vi "SendQuery.vi"(8 "error in (no error)":errorcluster, 11 "TCPComm in":refnum<class "TCPCommClass.lvclass">) -> (0 "error out":errorcluster, 3 "TCPComm out":refnum<class "TCPCommClass.lvclass">)   [LabVIEW 2013, in "TCPCommClass.lvclass"]
uses:
  TCPCommClass.lvclass
  TCPCommClass.lvclass/TCPCommClass.ctl
panel:
  in  "Initial byte timeout ms (1000)":i32=1000
  in  "old tcp":bool
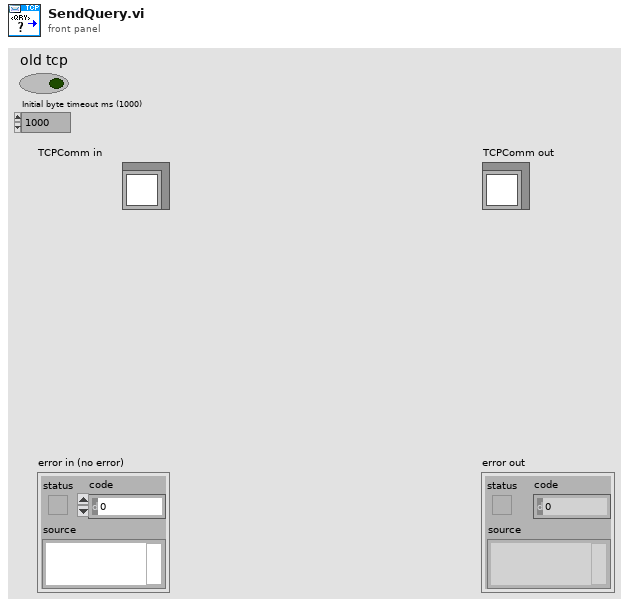
[diagram p1: front panel]
types:
  T1 = enum16{"Standard", "Buffered", "CRLF", "Immediate"}
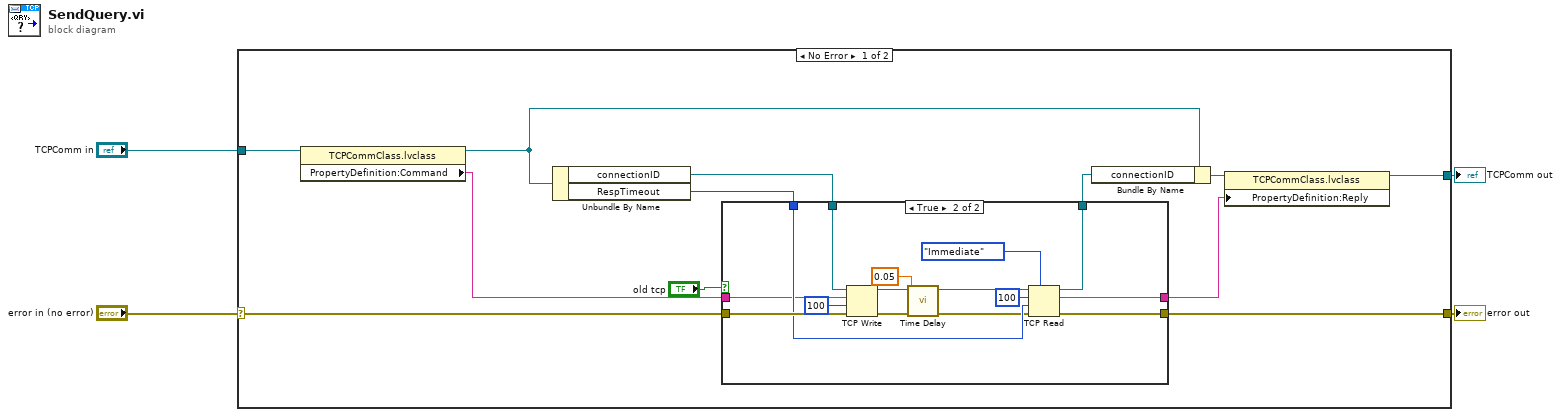
[diagram p0: block diagram]
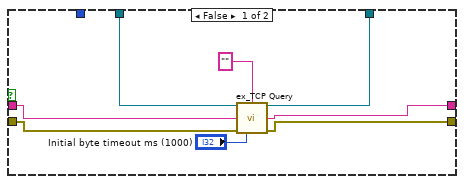
[diagram p2: hidden frame]
diagram:
  n1 = case shown="No Error" "error in (no error)" {
    selector: "error in (no error)" -> [w16 w40]
    tunnel: [w15 w40] -> w3
    tunnel: [w8 w39] -> w1
    tunnel: "TCPComm in" -> [w11 w39]
    frame No Error {
      n2 = property class="TCPCommClass.lvclass"(reference=w11) -> (reference out=w10:refnum<class "TCPCommClass.lvclass">, "PropertyDefinition:Command"=w6:string)  [unwired: 1 in, 1 out]
      n3 = Unbundle By Name(w10) -> ("connectionID"=w13:refnum<k5>, "RespTimeout"=w12:i32)
      n4 = case shown="True" "old tcp" {
        tunnel: w16 -> [w20 w34]
        tunnel: [w19 w33] -> w15
        tunnel: [w22 w32] -> w14
        tunnel: w13 -> [w23 w31]
        tunnel: w12 -> [_ w30]
        tunnel: [w18 w29] -> w7
        tunnel: w6 -> [w21 w28]
        frame False {
          n5 = call "ex_TCP Query.vi"("TCP Network Connection in"=w23, "Termination character"="", "Query string"=w21, "error in (no error)"=w20, "Initial byte timeout ms (1000)"="Initial byte timeout ms (1000)") -> ("TCP Network Connection out"=w22:refnum<k5>, "Message data out"=w18:string, "error out"=w19:errorcluster)  [unwired: 7 in, 1 out]
        }
        frame True {
          n6 = TCP Write(connection ID=w31, data in=w28, error in (no error)=w34, 9:100 ("bytes to read")) -> (connection ID out=w37:refnum<k5>, error out=w38:errorcluster)  [unwired: 1 out]
          n7 = call "Time Delay"("error in (no error)"=w38, "Delay Time (s)"=0.05) -> ("error out"=w26:errorcluster)  [unwired: 9 in]
          n8 = TCP Read(connection ID=w37, bytes to read=100, error in (no error)=w26, 7:T1."Immediate" ("mode (standard)"), 9:w30) -> (connection ID out=w32:refnum<k5>, data out=w29:string, error out=w33:errorcluster)
        }
      }
      n9 = Bundle By Name(cluster=w10, "connectionID"=w14) -> (w9:refnum<class "TCPCommClass.lvclass">)
      n10 = property class="TCPCommClass.lvclass"(reference=w9, "PropertyDefinition:Reply"=w7) -> (reference out=w8:refnum<class "TCPCommClass.lvclass">)  [unwired: 1 in, 1 out]
    }
    frame Error {
    }
  }
  "error out" <- w3
  "TCPComm out" <- w1
